vi "Get_data.vi"() -> (0 "EOF? and Error status":bool, 1 "Voltage output":dbl[][](graph), 2 "Analogue Binary":i16[][](array[numeric]), 3 "LDA Binary output":u16[][](array[numeric]), 4 "Block Timings":T1={"Started"=0.0, "Ended"=0.0, "Analogue Frequency Hz"=1000.0} {"Analogue Frequency Hz" format="%.2f"}, 5 "PWA Binary":i16[][](array[numeric]), 6 "Block Header":string)   [LabVIEW 2010]
uses:
  Controls/Block_start_and_end.ctl
  Controls/Board_Types.ctl
  Globals/Meas_global.vi
  Globals/LDA_meas_global_1.vi
  Globals/Dynamic_call_global.ph.vi
  Globals/Constants_global.vi
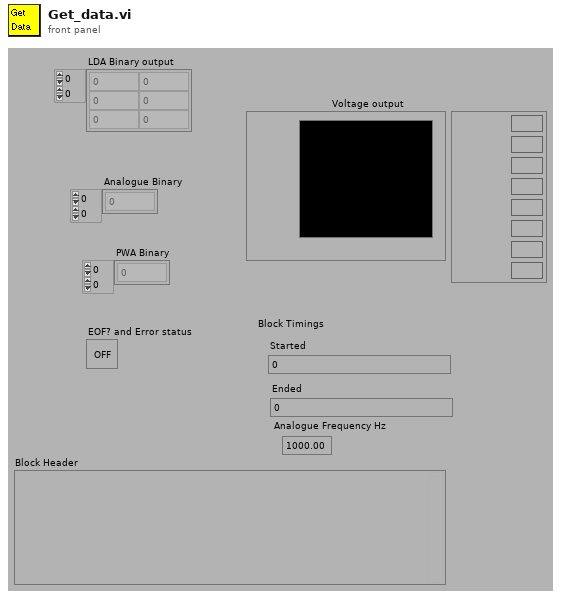
[diagram p1: front panel]
types:
  T1 = typedef "Block_start_and_end.ctl" = cluster{"Started":dbl, "Ended":dbl, "Analogue Frequency Hz":dbl}
  T2 = typedef "Board_Types.ctl" = enum16{"Simulate", "Local ADAM", "Server ADAM", "NI-DAQmx", "NI-DAQmxBase", "ADC488", "DT LV-link"}
  T3 = typedef "Post_Process.ctl" = enum16{"Take New Data", "Post Process Raw Data File"}
  T4 = typedef "PWA_Data.ctl" = enum16{"No PWA Data", "One Ch PWA"}
  T5 = typedef "BSA_Type.ctl" = enum16{"57N11", "BSA F60"}
  T6 = typedef "Ch_and_Spans.ctl" = cluster{"high limit (10V)":sgl, "low limit (-10V)":sgl, "Ch No":i16, "Var name":string, "Use Latest Calib":bool}
  T7 = cluster{"channel":string, "upper input limits":sgl, "lower input limits":sgl, "range":sgl, "polarity":u16, "gain":sgl, "coupling":u16, "input mode":u16, "scale multiplier":dbl, "scale offset":dbl}[]
  T8 = typedef "BSA_info_Cluster.ctl" = cluster{"GPIB Address":string, "No of Check Bytes":i32, "Extra Info":string, "COLOUR":u32, "Wavelength (nm)":dbl}
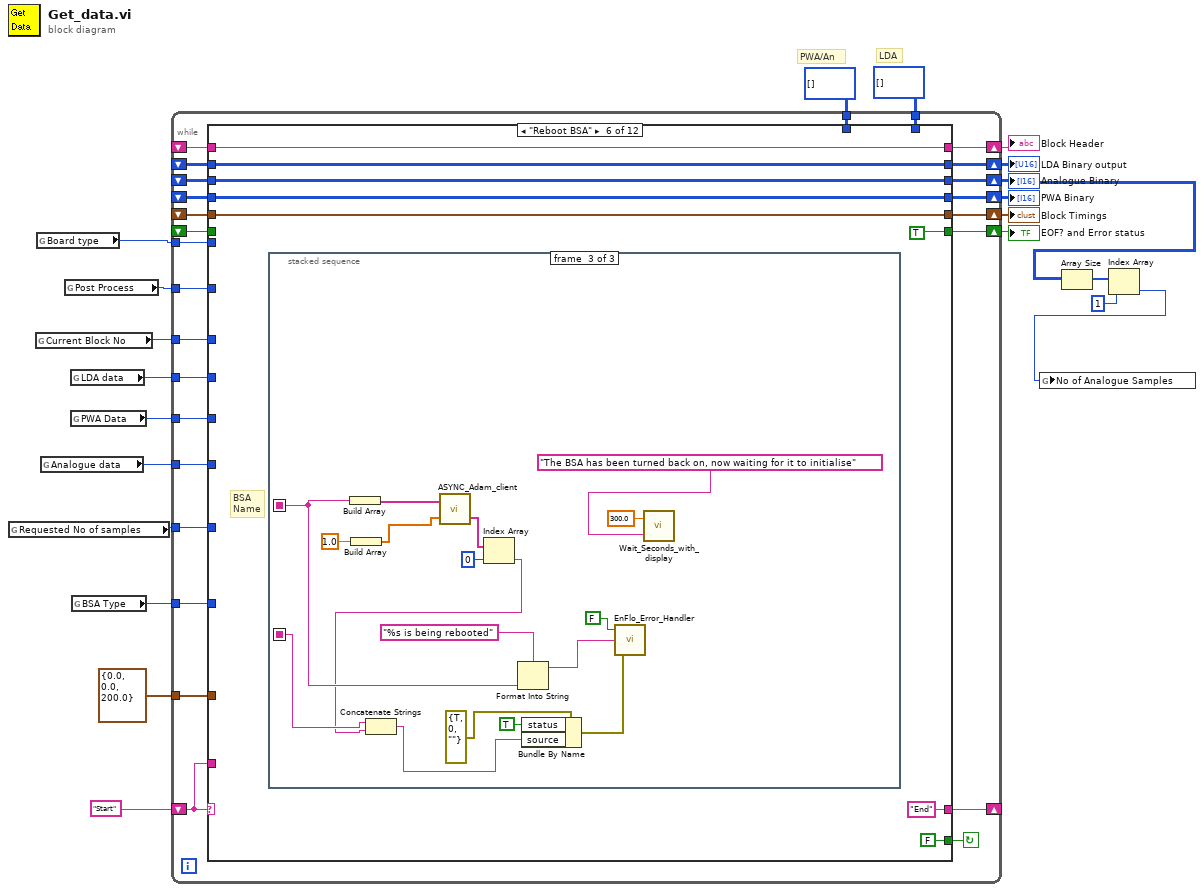
[diagram p0: block diagram]
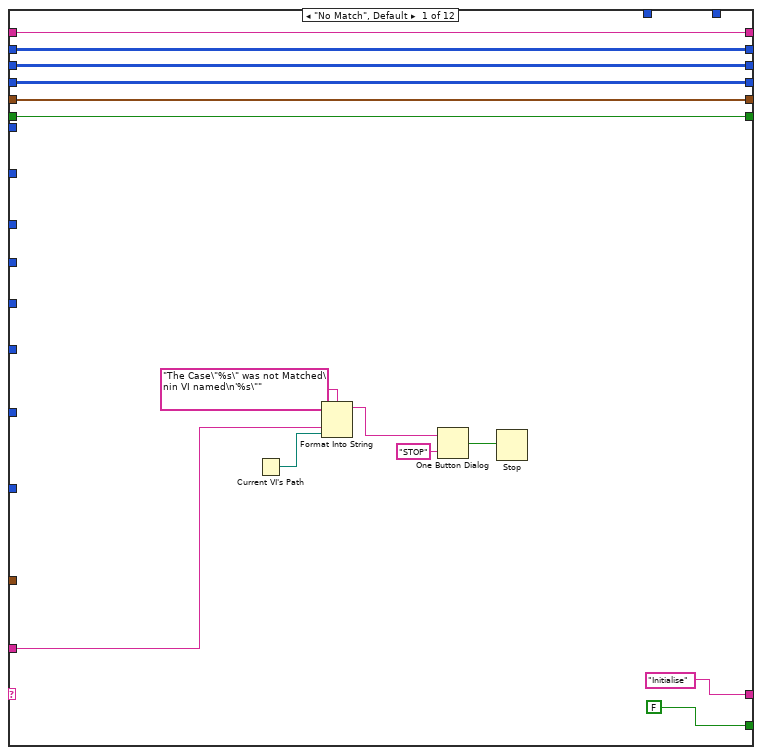
[diagram p2: hidden frame]
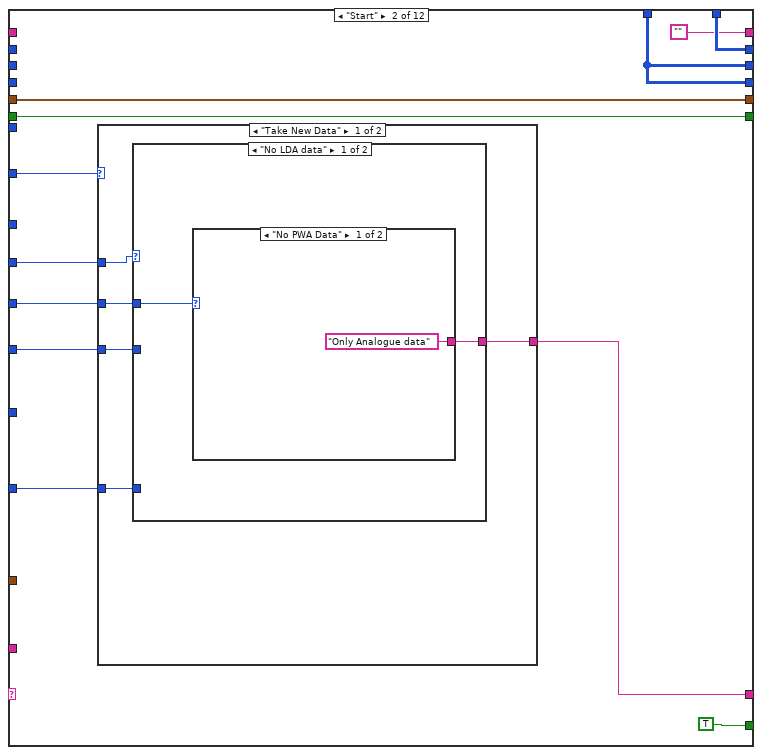
[diagram p3: hidden frame]
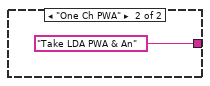
[diagram p4: hidden frame]
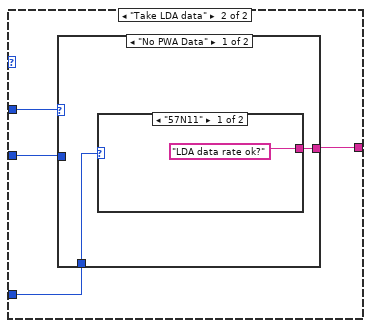
[diagram p5: hidden frame]
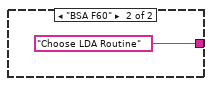
[diagram p6: hidden frame]
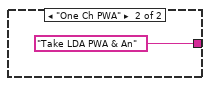
[diagram p7: hidden frame]
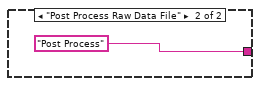
[diagram p8: hidden frame]
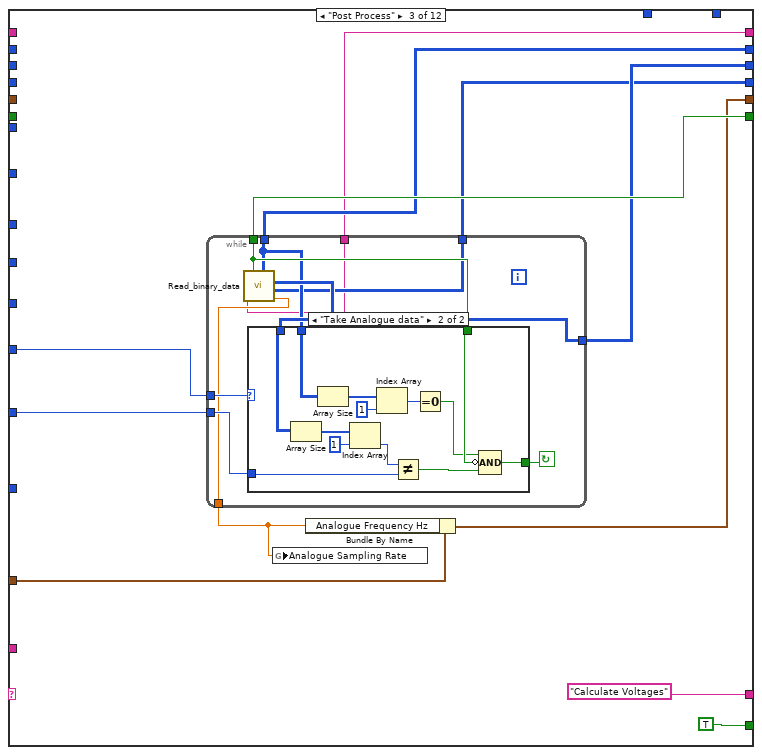
[diagram p9: hidden frame]
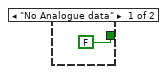
[diagram p10: hidden frame]
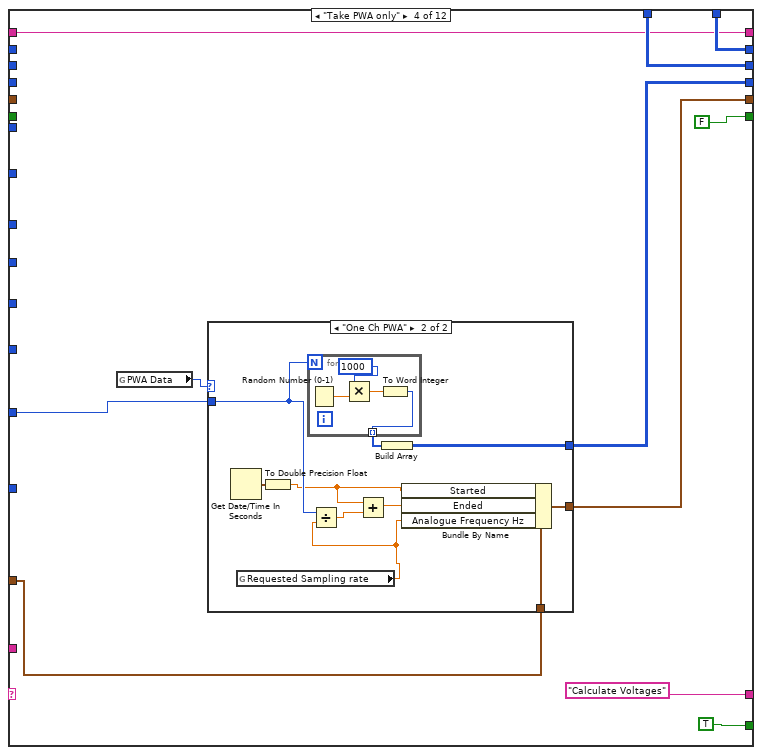
[diagram p11: hidden frame]
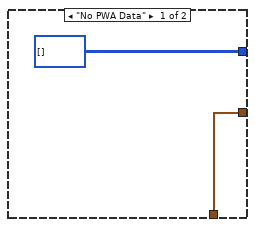
[diagram p12: hidden frame]
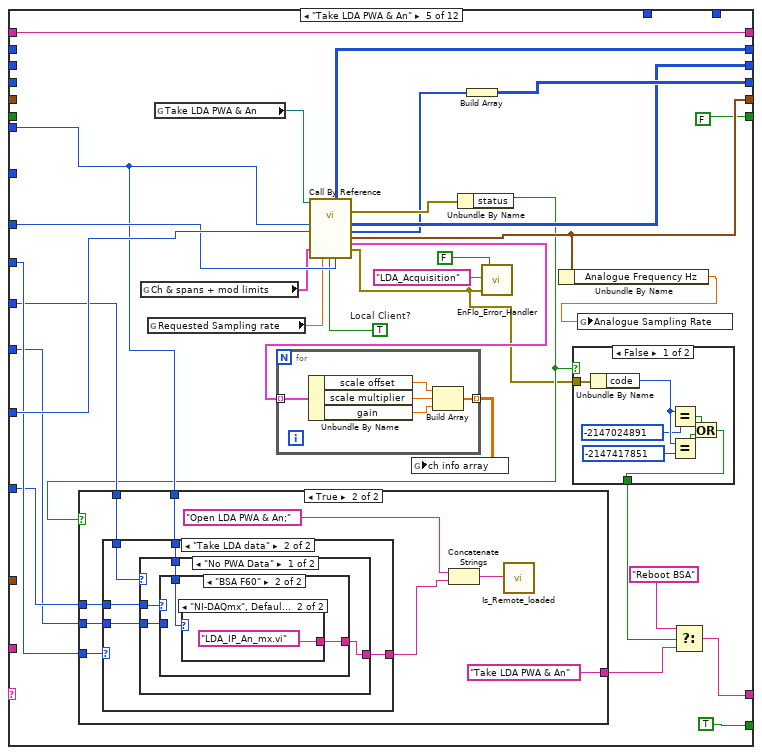
[diagram p13: hidden frame]
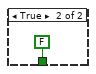
[diagram p14: hidden frame]
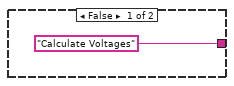
[diagram p15: hidden frame]
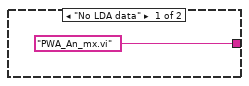
[diagram p16: hidden frame]
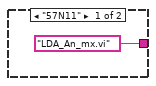
[diagram p17: hidden frame]
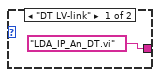
[diagram p18: hidden frame]
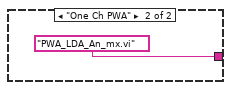
[diagram p19: hidden frame]
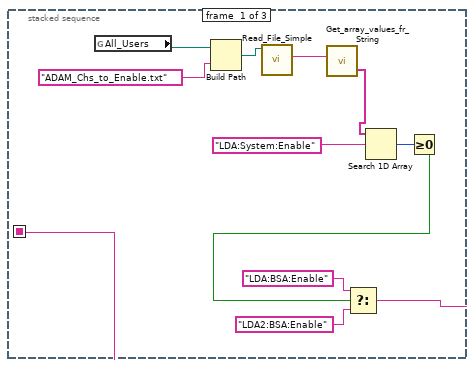
[diagram p20: hidden frame]
diagram:
  # "LDA"
  # "PWA/An"
  n1 = global read "Meas_global.vi" "Requested No of samples"() -> (w14:i32)
  n2 = global read "Meas_global.vi" "Current Block No"() -> (w13:i32)
  n3 = global read "Meas_global.vi" "Board type"() -> (w3:T2)
  n4 = global read "Meas_global.vi" "Analogue data"() -> (w12:enum16{"No Analogue data", "Take Analogue data"})
  n5 = global read "Meas_global.vi" "Post Process"() -> (w15:T3)
  n6 = global read "Meas_global.vi" "LDA data"() -> (w11:enum16{"No LDA data", "Take LDA data"})
  n7 = global read "Meas_global.vi" "PWA Data"() -> (w10:T4)
  n8 = global read "LDA_meas_global_1.vi" "BSA Type"() -> (w1:T5)
  n9 = while {
    shift-left: "Start" -> [w45]
    shift-right: [w46] -> _
    shift-right: [w44] -> w20
    shift-left: _ -> [w43]
    shift-right: [w42] -> w7
    shift-left: _ -> [w41]
    shift-right: [w40] -> w19
    shift-left: _ -> [w39]
    shift-right: [w38] -> w18
    shift-left: _ -> [w37]
    shift-right: [w36] -> w17
    shift-left: _ -> [w35]
    tunnel: T1 {"Started"=0.0, "Ended"=0.0, "Analogue Frequency Hz"=200.0} ("Block Timings") -> [w34]
    tunnel: w15 -> [w33]
    tunnel: w14 -> [w32]
    tunnel: w13 -> [w31]
    tunnel: w12 -> [w30]
    tunnel: w11 -> [w29]
    tunnel: w10 -> [w28]
    tunnel: u16[][] [] ("LDA Binary output") -> [w27]
    tunnel: i16[][] [] ("Analogue Binary output") -> [w26]
    tunnel: w3 -> [w25]
    tunnel: w1 -> [w24]
    shift-right: [w22] -> w2
    shift-left: _ -> [w23]
    stop <- w47 continue-if-true
    n10 = case shown="\"Reboot BSA\"" w45 {
      tunnel: [FALSE TRUE TRUE TRUE TRUE FALSE TRUE TRUE TRUE TRUE w422 FALSE] -> w47
      tunnel: ["Initialise" w69 "Calculate Voltages" "Calculate Voltages" w158 "End" ("t") "Calculate Voltages" w335 w385 "Calculate Voltages" "Save Raw Data" "End"] -> w46
      tunnel: w45 -> [w56 _ _ _ _ _ _ _ _ _ _ _]
      tunnel: [w53 w64 w99 w130 w180 w231 w273 w347 w393 w409 w429 w451] -> w44
      tunnel: w43 -> [w53 _ _ _ _ w231 _ w346 w393 _ w429 w451]
      tunnel: [w52 w65 w98 w129 w182 w230 w278 w344 w392 w408 w428 w450] -> w42
      tunnel: w41 -> [w52 _ _ _ _ w230 _ w345 w392 _ w428 w450]
      tunnel: [w51 w65 w95 w134 w183 w229 w272 w343 w391 w403 w426 w444] -> w40
      tunnel: w39 -> [w51 _ _ _ _ w229 _ w342 w391 _ w426 w444]
      tunnel: [w50 w72 w100 w133 w169 w228 w276 w341 w390 w407 w427 w447] -> w38
      tunnel: w37 -> [w50 w72 _ _ _ w228 _ w340 w390 _ w427 w447]
      tunnel: [w49 w71 w101 FALSE FALSE TRUE w277 w339 w389 w406 w425 w452] -> w36
      tunnel: w35 -> [w49 w71 _ _ _ _ _ w338 w389 _ w425 w452]
      tunnel: w34 -> [_ _ w102 w132 _ _ _ _ _ _ _ _]
      tunnel: w33 -> [_ w70 _ _ _ _ _ _ _ _ _ _]
      tunnel: w32 -> [_ _ w97 w135 w184 _ w280 _ _ _ _ _]
      tunnel: w31 -> [_ _ _ _ w181 _ w271 w350 _ _ _ w449]
      tunnel: w30 -> [_ w68 w96 _ w165 _ _ _ w387 _ _ _]
      tunnel: w29 -> [_ w67 _ _ w171 _ _ _ _ _ _ _]
      tunnel: w28 -> [_ w66 _ _ w170 _ _ _ _ _ _ _]
      tunnel: w27 -> [_ w64 _ w130 _ _ w273 _ _ _ _ _]
      tunnel: w26 -> [_ w65 _ w129 _ _ w272 _ _ w403 _ _]
      tunnel: w25 -> [_ _ _ _ w162 _ _ _ w388 _ _ _]
      tunnel: w24 -> [_ w63 _ _ w167 _ _ _ w383 _ _ _]
      tunnel: [w48 "" w93 w128 w166 w232 w270 w332 w384 w402 w420 w443] -> w22
      tunnel: w23 -> [w48 _ _ w128 w166 w232 _ w332 w384 w402 w420 w442]
      frame "No Match", Default {
        n11 = Current VI's Path() -> (path=w55:path)
        n12 = Format Into String(format string="The Case\"%s\" was not Matched\nin VI named\n'%s\"" ("Format String"), w56, w55) -> (resulting string=w59:string)  [unwired: 2 in, 1 out]
        n13 = One Button Dialog(message=w59, button name ("OK")="STOP") -> (true=w57:bool)
        n14 = Stop(stop? (T)=w57) -> ()
      }
      frame "Start" {
        n15 = case shown="\"Take New Data\"" w70 {
          tunnel: [w76 "Post Process"] -> w69
          tunnel: w68 -> [w78 _]
          tunnel: w67 -> [w77 _]
          tunnel: w66 -> [w75 _]
          tunnel: w63 -> [w74 _]
          frame "Take New Data" {
            n16 = case shown="\"No LDA data\"" w77 {
              tunnel: w78 -> [_ w84]
              tunnel: [w79 w86] -> w76
              tunnel: w75 -> [w80 w85]
              tunnel: w74 -> [_ w83]
              frame "No LDA data" {
                n17 = case shown="\"No PWA Data\"" w80 {
                  tunnel: ["Only Analogue data" "Take LDA PWA & An"] -> w79
                  frame "No PWA Data" {
                  }
                  frame "One Ch PWA" {
                  }
                }
              }
              frame "Take LDA data" {
                n18 = case shown="\"No PWA Data\"" w85 {
                  tunnel: [w87 "Take LDA PWA & An"] -> w86
                  tunnel: w84 -> [_ _]
                  tunnel: w83 -> [w88 _]
                  frame "No PWA Data" {
                    n19 = case shown="\"57N11\"" w88 {
                      tunnel: ["LDA data rate ok?" "Choose LDA Routine"] -> w87
                      frame "57N11" {
                      }
                      frame "BSA F60" {
                      }
                    }
                  }
                  frame "One Ch PWA" {
                  }
                }
              }
            }
          }
          frame "Post Process Raw Data File" {
          }
        }
      }
      frame "Post Process" {
        n20 = while {
          tunnel: [w107] -> w94
          tunnel: w96 -> [w109]
          tunnel: w97 -> [w110]
          tunnel: [w112] -> w101
          tunnel: [w108] -> w99
          tunnel: [w113] -> w98
          tunnel: [w106] -> w95
          tunnel: [w105] -> w93
          stop <- w111 continue-if-true
          n21 = call "Read_binary_data.vi"() -> ("Analogue Frequency Hz"=w107:dbl, "PWA Binary"=w106:i16[][], "Analogue Binary"=w113:i16[][], "LDA Binary output"=w108:u16[][], "EOF?"=w112:bool, "Block Header"=w105:string)  [unwired: 4 out]
          n22 = case shown="\"Take Analogue data\"" w109 {
            tunnel: w113 -> [_ w124]
            tunnel: w112 -> [_ w122]
            tunnel: [FALSE w121] -> w111
            tunnel: w110 -> [_ w120]
            tunnel: w108 -> [_ w117]
            frame "No Analogue data" {
            }
            frame "Take Analogue data" {
              n23 = Array Size(array=w124) -> (size(s)=w126:i32[])
              n24 = Array Size(array=w117) -> (size(s)=w119:i32[])
              n25 = Index Array(array=w126, index=1 ("Index")) -> (element=w125:i32)
              n26 = Index Array(array=w119, index=1 ("Index")) -> (element=w116:i32)
              n27 = Not Equal?(x=w125, y=w120) -> (x != y?=w123:bool)
              n28 = Equal To 0?(x=w116) -> (x = 0?=w115:bool)
              n29 = Compound Arithmetic op=AND(w115, invert w122, w123) -> (w121:bool)
            }
          }
        }
        n30 = global write "Meas_global.vi" "Analogue Sampling Rate"(w94) -> ()
        n31 = Bundle By Name(cluster=w102, "Analogue Frequency Hz"=w94) -> (w100:T1)
      }
      frame "Take PWA only" {
        n32 = global read "Meas_global.vi" "PWA Data"() -> (w136:T4)
        n33 = case shown="\"One Ch PWA\"" w136 {
          tunnel: w135 -> [_ w147]
          tunnel: [i16[][] [] w149] -> w134
          tunnel: [w139 w143] -> w133
          tunnel: w132 -> [w139 w142]
          frame "No PWA Data" {
          }
          frame "One Ch PWA" {
            n34 = Get Date/Time In Seconds() -> (seconds since 1Jan1904=w148:timestamp)
            n35 = global read "Meas_global.vi" "Requested Sampling rate"() -> (w146:dbl)
            n36 = To Double Precision Float(number=w148) -> (double precision float=w144:dbl)
            n37 = for {
              N: w147 -> [_]
              tunnel: [w151] -> w150 mode=indexing
              n38 = Random Number (0-1)() -> (number: 0 to 1=w154:dbl)
              n39 = Multiply(x=1000, y=w154) -> (x*y=w152:dbl)
              n40 = To Word Integer(number=w152) -> (16bit integer=w151:i16)
            }
            n41 = Divide(x=w147, y=w146) -> (x/y=w145:dbl)
            n42 = Add(x=w144, y=w145) -> (x+y=w141:dbl)
            n43 = Build Array(w150) -> (w149:i16[][])
            n44 = Bundle By Name(cluster=w142, "Started"=w144, "Ended"=w141, "Analogue Frequency Hz"=w146) -> (w143:T1)
          }
        }
      }
      frame "Take LDA PWA & An" {
        w176 = TRUE  # Local Client?
        n45 = global read "Meas_global.vi" "Ch & spans + mod limits"() -> (w179:T6[])
        n46 = global read "Meas_global.vi" "Requested Sampling rate"() -> (w175:dbl)
        n47 = global read "Dynamic_call_global.ph.vi" "Take LDA PWA & An"() -> (w174:refnum<vi>)
        n48 = call-by-ref "?"(reference=w174, "Board type"=w162, "No of LDA samples"=w184, "Ch & spans"=w179, "LDA Sampling rate (Hz)"=w175, "Local Client?"=w176, "Current Block No"=w181) -> (error out=w173:errorcluster, "LDA Binary output"=w180:u16[][], "I16 Analogue data block"=w182:i16[][], "I16 TOF block (mu.s)"=w172:i16[], "Block Timings"=w169:T1, "group channel settings"=w178:T7, 15:"error out"=w160:errorcluster)  [unwired: 5 in, 1 out]
        n49 = for {
          tunnel: w178 -> [w224] mode=indexing
          tunnel: [w220] -> w177 mode=indexing
          n50 = Unbundle By Name(w224) -> ("scale offset"=w223:dbl, "scale multiplier"=w222:dbl, "gain"=w221:sgl)
          n51 = Build Array(w223, w222, w221) -> (w220:dbl[])
        }
        n52 = global write "Meas_global.vi" "ch info array"(w177) -> ()
        n53 = Unbundle By Name(w173) -> ("status"=w161:bool)
        n54 = case shown="True" w161 {
          tunnel: ["Calculate Voltages" "Take LDA PWA & An"] -> w157
          tunnel: w171 -> [_ w199]
          tunnel: w170 -> [_ w198]
          tunnel: w167 -> [_ w197]
          tunnel: w165 -> [_ w196]
          tunnel: w162 -> [_ w195]
          frame False {
          }
          frame True {
            n55 = case shown="\"Take LDA data\"" w199 {
              tunnel: ["PWA_An_mx.vi" ("name or relative path") w209] -> w200
              tunnel: w198 -> [_ w208]
              tunnel: w197 -> [_ w207]
              tunnel: w196 -> [_ w206]
              tunnel: w195 -> [_ w205]
              frame "No LDA data" {
              }
              frame "Take LDA data" {
                n56 = case shown="\"No PWA Data\"" w208 {
                  tunnel: [w212 "PWA_LDA_An_mx.vi" ("name or relative path")] -> w209
                  tunnel: w207 -> [w213 _]
                  tunnel: w206 -> [w211 _]
                  tunnel: w205 -> [w210 _]
                  frame "No PWA Data" {
                    n57 = case shown="\"BSA F60\"" w213 {
                      tunnel: ["LDA_An_mx.vi" ("name or relative path") w216] -> w212
                      tunnel: w211 -> [_ _]
                      tunnel: w210 -> [_ w215]
                      frame "57N11" {
                      }
                      frame "BSA F60" {
                        n58 = case shown="\"NI-DAQmx\", Default" w215 {
                          tunnel: ["LDA_IP_An_DT.vi" ("name or relative path") "LDA_IP_An_mx.vi" ("name or relative path")] -> w216
                          frame "DT LV-link" {
                          }
                          frame "NI-DAQmx", Default {
                          }
                        }
                      }
                    }
                  }
                  frame "One Ch PWA" {
                  }
                }
              }
            }
            n59 = Concatenate Strings("Open LDA PWA & An;", w200) -> (w201:string)
            n60 = call "Is_Remote_loaded.vi"("Sub VI to call"=w201) -> ()
          }
        }
        n61 = Build Array(w172) -> (w183:i16[][])
        n62 = call "EnFlo_Error_Handler.vi"("error in (no error)"=w160, "Error Type"="LDA_Acquisition", "Dialog Box (T)"=FALSE) -> ()  [unwired: 3 out]
        n63 = Unbundle By Name(w169) -> ("Analogue Frequency Hz"=w168:dbl)
        n64 = case shown="False" w161 {
          tunnel: w160 -> [w192 _]
          tunnel: [w186 FALSE] -> w159
          frame False {
            n65 = Unbundle By Name(w192) -> ("code"=w191:i32)
            n66 = Equal?(x=w191, y=-2147024891) -> (x = y?=w188:bool)
            n67 = Equal?(x=w191, y=-2147417851) -> (x = y?=w187:bool)
            n68 = Or(x=w188, y=w187) -> (x .or. y?=w186:bool)
          }
          frame True {
          }
        }
        n69 = global write "Meas_global.vi" "Analogue Sampling Rate"(w168) -> ()
        n70 = Select(t="Reboot BSA", s=w159, f=w157) -> (s? t:f=w158:string)
      }
      frame "Reboot BSA" {
        # "BSA\nName"
        n71 = stacked-sequence {
          seq-local: [w233 _ _] -> [_ w250 w264]
          seq-local: [_ w244 _] -> [_ _ w255]
          frame #0 {
            n72 = global read "Constants_global.vi" "All_Users"() -> (w243:path)
            n73 = Build Path(base path=w243, name or relative path="ADAM_Chs_to_Enable.txt") -> (appended path=w242:path)
            n74 = call "Read_File_Simple.vi"("Filename"=w242) -> ("string"=w241:string)  [unwired: 2 in, 7 out]
            n75 = call "Get_array_values_fr_String.vi"("String Value"=w241) -> ("String array"=w239:string[])  [unwired: 1 out]
            n76 = Search 1D Array(1D array=w239, element="LDA:System:Enable") -> (index of element=w237:i32)  [unwired: 1 in]
            n77 = Greater Or Equal To 0?(x=w237) -> (x >= 0?=w234:bool)
            n78 = Select(t="LDA:BSA:Enable", s=w234, f="LDA2:BSA:Enable") -> (s? t:f=w233:string)
          }
          frame #1 {
            n79 = Build Array(w250) -> (w249:string[])
            n80 = Build Array(0.0) -> (w251:dbl[])
            n81 = call "ASYNC_Adam_client.vi"("Values"=w251, "Channel Names"=w249) -> ("Scan Comments"=w248:string[])  [unwired: 1 out]
            n82 = Index Array(array=w248, index=0) -> (element=w244:string)
            n83 = call "Wait_Seconds_with_display.vi"("Message"="The BSA has been turned off to reboot it ", "Seconds to wait"=15.0) -> ()  [unwired: 1 in, 1 out]
          }
          frame #2 {
            n84 = Build Array(w264) -> (w263:string[])
            n85 = Build Array(1.0) -> (w268:dbl[])
            n86 = call "ASYNC_Adam_client.vi"("Values"=w268, "Channel Names"=w263) -> ("Scan Comments"=w259:string[])  [unwired: 1 out]
            n87 = Index Array(array=w259, index=0) -> (element=w254:string)
            n88 = Concatenate Strings(w255, w254) -> (w253:string)
            n89 = Format Into String(format string="%s is being rebooted" ("Error Type"), w264) -> (resulting string=w265:string)  [unwired: 2 in, 1 out]
            n90 = Bundle By Name(cluster=errorcluster {"status"=TRUE, "code"=0, "source"=""} ("error in (no error)"), "status"=TRUE, "source"=w253) -> (w261:errorcluster)
            n91 = call "EnFlo_Error_Handler.vi"("error in (no error)"=w261, "Error Type"=w265, "Dialog Box (T)"=FALSE) -> ()  [unwired: 3 out]
            n92 = call "Wait_Seconds_with_display.vi"("Message"="The BSA has been turned back on, now waiting for it to initialise", "Seconds to wait"=300.0) -> ()  [unwired: 1 in, 1 out]
          }
        }
      }
      frame "Only Analogue data" {
        n93 = global read "Meas_global.vi" "Board type"() -> (w282:T2)
        n94 = Not Equal?(x=w282, y=Board_Types."Simulate" ("Board type")) -> (x != y?=w279:bool)
        n95 = while {
          tunnel: w280 -> [w291]
          tunnel: w279 -> [w290]
          tunnel: [w289] -> w278
          tunnel: [w287] -> w277
          tunnel: [w286] -> w276
          tunnel: w271 -> [w284]
          tunnel: [w283] -> w270
          i -> [w285]
          stop <- w288 continue-if-true
          n96 = stacked-sequence {
            seq-local: [w300 _ _] -> [_ w317 w318]
            seq-local: [_ w308 _] -> [_ _ w320]
            seq-local: [w295 _ _] -> [_ w315 _]
            tunnel: [_ w305 _] -> w288
            tunnel: [w301 _ _] -> w289
            tunnel: w291 -> [_ w316 w319]
            tunnel: [w299 _ _] -> w286
            tunnel: [w293 _ _] -> w287
            tunnel: w290 -> [_ w312 _]
            tunnel: w285 -> [_ w311 _]
            tunnel: w284 -> [_ w304 _]
            tunnel: [w292 _ _] -> w283
            frame #0 {
              n97 = call "Acquire_Data.vi"() -> ("Binary output"=w301:i16[][], "Block Timings"=w299:T1, "Add to Block Header"=w292:string, "error out"=w294:errorcluster)  [unwired: 12 out]
              n98 = Array Size(array=w301) -> (size(s)=w298:i32[])
              n99 = Index Array(array=w298, index=0) -> (element=w296:i32)
              n100 = Index Array(array=w298, index=1 ("Index")) -> (element=w300:i32)
              n101 = Greater Than 0?(x=w296) -> (x > 0?=w295:bool)
              n102 = Unbundle By Name(w294) -> ("status"=w293:bool)
            }
            frame #1 {
              n103 = Not Equal?(x=w316, y=w317) -> (x != y?=w314:bool)
              n104 = Equal To 0?(x=w304) -> (x = 0?=w303:bool)
              n105 = Compound Arithmetic op=AND(w314, w312) -> (w313:bool)
              n106 = And(x=w315, y=w313) -> (x .and. y?=w308:bool)
              n107 = call "Pause_Acquisition.vi"() -> ("Paused"=w307:bool)
              n108 = Less?(x=w311, y=2) -> (x < y?=w309:bool)
              n109 = Compound Arithmetic op=AND(w303, w308, w309) -> (w306:bool)
              n110 = Or(x=w307, y=w306) -> (x .or. y?=w305:bool)
            }
            frame #2 {
              n111 = case shown="True" w320 {
                tunnel: w319 -> [_ w328]
                tunnel: w318 -> [_ w327]
                frame False {
                }
                frame True {
                  w329 = FALSE  # Dialog Box
                  n112 = Format Into String(format string="Desired No of samples %d, Achieved %d" ("Format String"), w328, w327) -> (resulting string=w322:string)  [unwired: 2 in, 1 out]
                  n113 = global read "Meas_global.vi" "Extra Comments"() -> (w323:string)
                  n114 = Concatenate Strings(w323, w322) -> (w321:string)
                  n115 = global write "Meas_global.vi" "Extra Comments"(w321) -> ()
                  n116 = Bundle By Name(cluster=errorcluster {"status"=FALSE, "code"=0, "source"=""} ("error in (no error)"), "status"=TRUE ("Bundle Element"), "source"=w322) -> (w330:errorcluster)
                  n117 = call "EnFlo_Error_Handler.vi"("error in (no error)"=w330, "Error Type"="No of Samples Error", "Dialog Box (T)"=w329) -> ()  [unwired: 3 out]
                }
              }
            }
          }
        }
      }
      frame "LDA data rate ok?" {
        n118 = while {
          tunnel: [w373] -> w349 mode=indexing
          tunnel: [w375] -> w336
          i -> [w378]
          stop <- w374 continue-if-true
          n119 = global read "LDA_meas_global_1.vi" "BSA1 info"() -> (w381:T8)
          n120 = Unbundle By Name(w381) -> ("GPIB Address"=w380:string)
          n121 = Less?(x=w378, y=8) -> (x < y?=w376:bool)
          n122 = call "data_rate.vi"("GPIB address"=w380) -> ("Data rate (Hz)"=w373:dbl)
          n123 = Greater?(x=w373, y=5.0) -> (0:w375:bool)
          n124 = Compound Arithmetic op=AND(invert w375, w376) -> (w374:bool)
          n125 = case shown="True" w374 {
            frame False {
            }
            frame True {
              n126 = Wait Until Next ms Multiple(millisecond multiple=u32 1000) -> ()  [unwired: 1 out]
            }
          }
        }
        n127 = Array Max & Min(array=w349) -> (max value=w348:dbl)  [unwired: 3 out]
        n128 = case shown="True" w336 {
          tunnel: w350 -> [_ w368]
          tunnel: w348 -> [w352 w367]
          tunnel: [u16[][] [] ("LDA Binary output") w366] -> w347
          tunnel: w346 -> [_ w366]
          tunnel: w345 -> [_ w365]
          tunnel: [i16[][] [] ("Binary output") w365] -> w344
          tunnel: [w359 w364] -> w343
          tunnel: w342 -> [w359 w364]
          tunnel: [T1 {"Started"=0.0, "Ended"=0.0, "Analogue Frequency Hz"=200.0} ("Block Timings") w363] -> w341
          tunnel: w340 -> [_ w363]
          tunnel: [TRUE w362] -> w339
          tunnel: w338 -> [_ w362]
          frame False {
            n129 = Number To Fractional String(number=w352, precision (6)=1) -> (F-format string=w354:string)  [unwired: 2 out]
            n130 = Concatenate Strings("BSA data rate is ", w354, " Hz.") -> (w357:string)
            n131 = global write "Meas_global.vi" "BSA data rate string"(w357) -> ()
          }
          frame True {
            n132 = Greater?(x=w368, y=1) -> (0:w370:bool)
            n133 = global read "Meas_global.vi" "LDA frequency"() -> (w372:dbl)
            n134 = Select(t=w372, s=w370, f=w367) -> (s? t:f=w369:dbl)
            n135 = global write "Meas_global.vi" "Actual Sampling rate (Hz)"(w369) -> ()
          }
        }
        n136 = Select(t="Choose LDA Routine", s=w336, f="Calculate Voltages") -> (s? t:f=w335:string)
      }
      frame "Choose LDA Routine" {
        n137 = case shown="\"Take Analogue data\"" w387 {
          tunnel: [w395 w399] -> w385
          tunnel: w388 -> [_ w398]
          tunnel: w383 -> [w394 _]
          frame "No Analogue data" {
            n138 = case shown="\"BSA F60\"" w394 {
              tunnel: ["Take LDA+Analogue data" "Take LDA PWA & An"] -> w395
              frame "57N11" {
              }
              frame "BSA F60" {
              }
            }
          }
          frame "Take Analogue data" {
            n139 = case shown="\"NI-DAQmx\", Default" w398 {
              tunnel: ["Take LDA PWA & An" "Take LDA+Analogue data"] -> w399
              frame "NI-DAQmx", Default {
              }
              frame "ADC488" {
              }
            }
          }
        }
      }
      frame "Take LDA+Analogue data" {
        n140 = while {
          tunnel: [w410] -> w406
          tunnel: [w411] -> w407
          tunnel: [w413] -> w409
          tunnel: [w412] -> w408
          i -> [w414]
          stop <- w415 continue-if-true
          n141 = Less?(x=w414, y=1) -> (x < y?=w418:bool)
          n142 = call "Get_LDA_+_An_data.vi"("Try number"=w414) -> ("LDA Binary output"=w413:u16[][], "Analogue Binary output"=w412:i16[][], "Block Timings"=w411:T1, "Repeat Block"=w410:bool)
          n143 = And(x=w410, y=w418) -> (x .and. y?=w417:bool)
          n144 = call "Pause_Acquisition.vi"() -> ("Paused"=w416:bool)
          n145 = Or(x=w416, y=w417) -> (x .or. y?=w415:bool)
        }
      }
      frame "Calculate Voltages" {
        n146 = global read "Meas_global.vi" "ch info array"() -> (w430:dbl[][])
        n147 = global read "Meas_global.vi" "Raw data option"() -> (w424:enum16{"Save raw data", "Raw data not saved"})
        n148 = for {
          tunnel: [w433] -> w421 mode=indexing
          tunnel: w428 -> [w440] mode=indexing
          tunnel: w430 -> [w436] mode=indexing
          n149 = To Double Precision Float(number=w440) -> (double precision float=w439:dbl[])
          n150 = Index Array(array=w436, index=0) -> (element=w435:dbl)
          n151 = Index Array(array=w436, index=1) -> (element=w434:dbl)
          n152 = Multiply(x=w439, y=w434) -> (x*y=w441:dbl[])
          n153 = Add(x=w435, y=w441) -> (x+y=w433:dbl[])
        }
        "Voltage output" <- w421
        n154 = case shown="\"Raw data not saved\"" w424 {
          tunnel: [TRUE FALSE] -> w422
          frame "Save raw data" {
          }
          frame "Raw data not saved" {
          }
        }
      }
      frame "Save Raw Data" {
        n155 = Greater Than 0?(x=w449) -> (x > 0?=w448:bool)
        n156 = call "Save_Raw_data.vi"("Add to Block Header"=w442, "PWA Binary"=w444, "Analogue Binary"=w450, "append to file? (new file:F)"=w448, "Block Timings"=w447, "LDA Binary"=w451) -> ("Block Header"=w443:string)  [unwired: 3 in]
      }
    }
  }
  "EOF? and Error status" <- w17
  "LDA Binary output" <- w20
  "Analogue Binary" <- w7
  "PWA Binary" <- w19
  "Block Timings" <- w18
  "Block Header" <- w2
  n157 = Array Size(array=w7) -> (size(s)=w6:i32[])
  n158 = Index Array(array=w6, index=1) -> (element=w4:i32)
  n159 = global write "Meas_global.vi" "No of Analogue Samples"(w4) -> ()
